vi "Configure Temperature 4Wire RTD Type.vi"(8 "error in (no error)":errorcluster, 9 "4 Wire RTD Type":u16(ring) items=["PT100", "D100", "F100", "PT385", "PT3916", "User-specified"], 11 "VISA resource name":refnum<visa-resource-name>) -> (0 "error out":errorcluster, 3 "VISA resource name out":refnum<visa-resource-name>)   [LabVIEW 2018, in "Keithley DMM7512.lvlib"]
doc: "This VI defines the type of four-wire RTD that is being used."
uses:
  <instrlib>/Keithley DMM7512/Keithley DMM7512.lvlib
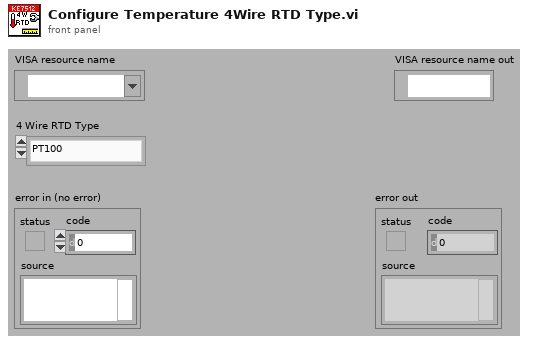
[diagram p1: front panel]
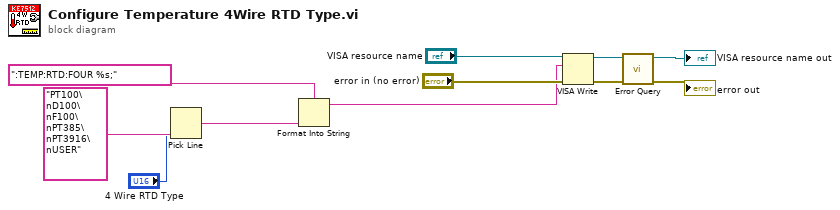
[diagram p0: block diagram]
diagram:
  n1 = Pick Line(multi-line string="PT100\nD100\nF100\nPT385\nPT3916\nUSER", line index="4 Wire RTD Type") -> (output string=w7:string)  [unwired: 1 in]
  n2 = Format Into String(format string=":TEMP:RTD:FOUR %s;", w7) -> (resulting string=w1:string)  [unwired: 2 in, 1 out]
  n3 = VISA Write(VISA resource name="VISA resource name", write buffer=w1, error in (no error)="error in (no error)") -> (VISA resource name out=w6:refnum<visa-resource-name>, error out=w5:errorcluster)  [unwired: 1 out]
  n4 = call <instrlib>:"Error Query.vi"("error in (no error)"=w5, "VISA resource name"=w6) -> ("error out"=→"error out":errorcluster, "VISA resource name out"=→"VISA resource name out":refnum<visa-resource-name>)  [unwired: 6 in, 2 out]
